vi "Initialize Actor.vi"(7 "Host Name":string, 8 "error in (no error)":errorcluster, 9 "Actor Name":string, 10 "Message Broker Interface":refnum<class "Message Broker Interface.lvclass">, 11 "Replay in":refnum<class "Replay.lvclass">) -> (0 "error out":errorcluster, 3 "Replay out":refnum<class "Replay.lvclass">)   [LabVIEW 2016, in "CLD Exam - ATM.lvlib" / "Replay.lvclass"]
uses:
  Replay.lvclass
  Mediator/Classes/Message Broker Interface/Message Broker Interface.lvclass
  Replay.lvclass/Replay.ctl
  Mediator/Classes/Message Transport Event/Message Transport Event.lvclass
  D:/Repos/Stream/software/Mediator/Classes/Message Transport Interface/Message Transport Interface.lvclass
  Mediator/Classes/Mediated Synchronous Actor/Mediated Synchronous Actor.lvclass
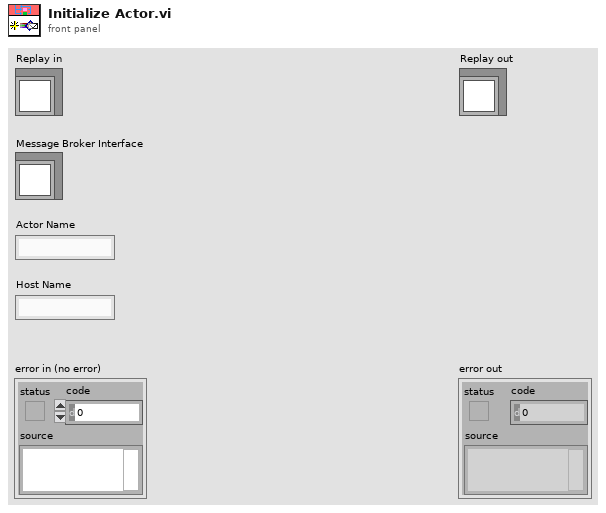
[diagram p1: front panel]
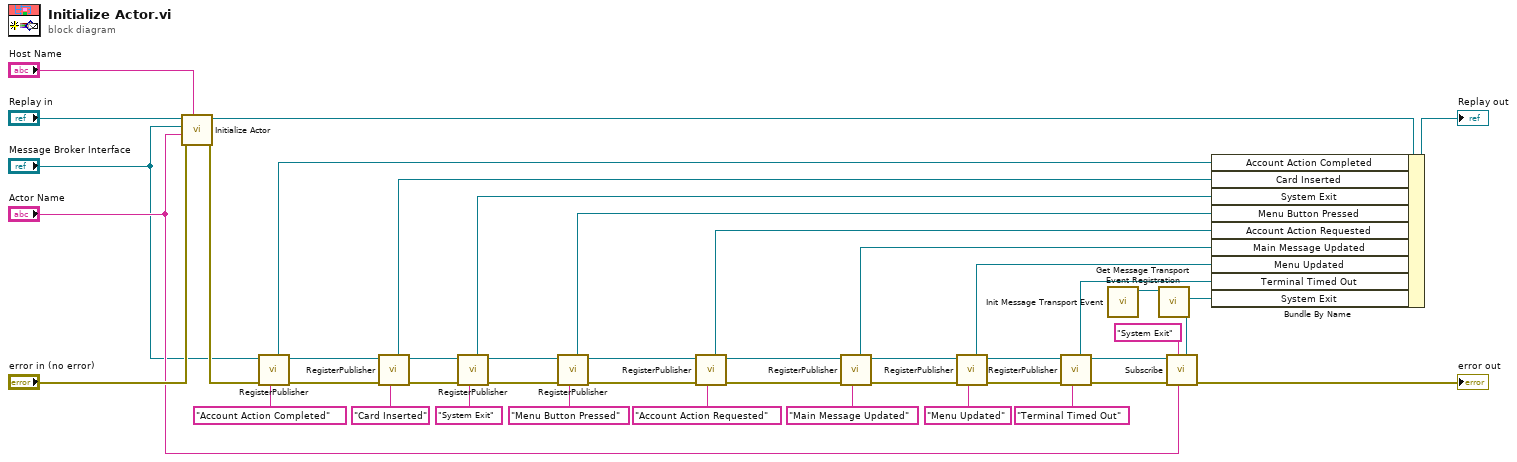
[diagram p0: block diagram]
diagram:
  n1 = call-parent "Initialize Actor.vi"("Host Name"="Host Name", "error in (no error)"="error in (no error)", "Actor Name"="Actor Name", "Message Broker Interface"="Message Broker Interface", "Mediated Synchronous Actor in"="Replay in") -> ("error out"=w33:errorcluster, "Mediated Synchronous Actor out"=w42:refnum<class "Replay.lvclass">)  [unwired: 5 in]
  n2 = call-dynamic "RegisterPublisher.vi"("Topic Name"="Account Action Completed", "error in (no error)"=w33, "Message Broker Interface in"="Message Broker Interface") -> ("error out"=w28:errorcluster, "Message Broker Interface out"=w29:refnum<class "Message Broker Interface.lvclass">, "Transport"=w31:refnum<class "Message Transport Queue.lvclass">)  [unwired: 4 in, 2 out]
  n3 = call-dynamic "RegisterPublisher.vi"("Topic Name"="Card Inserted", "error in (no error)"=w28, "Message Broker Interface in"=w29) -> ("error out"=w24:errorcluster, "Message Broker Interface out"=w25:refnum<class "Message Broker Interface.lvclass">, "Transport"=w26:refnum<class "Message Transport Queue.lvclass">)  [unwired: 4 in, 2 out]
  n4 = call-dynamic "RegisterPublisher.vi"("Topic Name"="System Exit", "error in (no error)"=w24, "Message Broker Interface in"=w25) -> ("error out"=w20:errorcluster, "Message Broker Interface out"=w21:refnum<class "Message Broker Interface.lvclass">, "Transport"=w23:refnum<class "Message Transport Queue.lvclass">)  [unwired: 4 in, 2 out]
  n5 = call-dynamic "RegisterPublisher.vi"("Topic Name"="Menu Button Pressed", "error in (no error)"=w20, "Message Broker Interface in"=w21) -> ("error out"=w16:errorcluster, "Message Broker Interface out"=w17:refnum<class "Message Broker Interface.lvclass">, "Transport"=w19:refnum<class "Message Transport Queue.lvclass">)  [unwired: 4 in, 2 out]
  n6 = call-dynamic "RegisterPublisher.vi"("Topic Name"="Account Action Requested", "error in (no error)"=w16, "Message Broker Interface in"=w17) -> ("error out"=w12:errorcluster, "Message Broker Interface out"=w13:refnum<class "Message Broker Interface.lvclass">, "Transport"=w15:refnum<class "Message Transport Queue.lvclass">)  [unwired: 4 in, 2 out]
  n7 = call-dynamic "RegisterPublisher.vi"("Topic Name"="Main Message Updated", "error in (no error)"=w12, "Message Broker Interface in"=w13) -> ("error out"=w8:errorcluster, "Message Broker Interface out"=w9:refnum<class "Message Broker Interface.lvclass">, "Transport"=w11:refnum<class "Message Transport Queue.lvclass">)  [unwired: 4 in, 2 out]
  n8 = call-dynamic "RegisterPublisher.vi"("Topic Name"="Menu Updated", "error in (no error)"=w8, "Message Broker Interface in"=w9) -> ("error out"=w2:errorcluster, "Message Broker Interface out"=w4:refnum<class "Message Broker Interface.lvclass">, "Transport"=w7:refnum<class "Message Transport Queue.lvclass">)  [unwired: 4 in, 2 out]
  n9 = call-dynamic "RegisterPublisher.vi"("Topic Name"="Terminal Timed Out", "error in (no error)"=w2, "Message Broker Interface in"=w4) -> ("error out"=w1:errorcluster, "Message Broker Interface out"=w3:refnum<class "Message Broker Interface.lvclass">, "Transport"=w5:refnum<class "Message Transport Queue.lvclass">)  [unwired: 4 in, 2 out]
  n10 = call "Init Message Transport Event.vi"() -> ("Message Transport Event out"=w38:refnum<class "Message Transport Event.lvclass">)  [unwired: 10 in, 1 out]
  n11 = call "Get Message Transport Event Registration.vi"("Message Transport Event in"=w38) -> ("Event Registration Refnum"=w36:refnum<event-registration>, "Message Transport Event out"=w39:refnum<class "Message Transport Event.lvclass">)  [unwired: 7 in, 2 out]
  n12 = call-dynamic "Subscribe.vi"("Message Transport Interface"=w39, "Subscriber Name"="Actor Name", "Topic Name"="System Exit", "error in (no error)"=w1, "Message Broker Interface in"=w3) -> ("error out"=→"error out":errorcluster)  [unwired: 4 in, 2 out]
  n13 = Bundle By Name(cluster=w42, "Account Action Completed"=w31, "Card Inserted"=w26, "System Exit"=w23, "Menu Button Pressed"=w19, "Account Action Requested"=w15, "Main Message Updated"=w11, "Menu Updated"=w7, "Terminal Timed Out"=w5, "System Exit"=w36) -> (→"Replay out":refnum<class "Replay.lvclass">)
